vi "ReleaseLock.vi"(7 "Key":T1, 8 "error in (no error)":errorcluster, 11 "Object in":refnum<class "OpenG_Reference_Object.lvclass">) -> (0 "error out":errorcluster, 3 "Object out":refnum<class "OpenG_Reference_Object.lvclass">)   [LabVIEW 2015, in "OpenG_Reference_Object.lvclass"]
doc: "Releases a locked object to allow other parallel threads to access the object. Proper key is required to unlock an object."
uses:
  <userlib>/_OpenG.lib/openg_object/openg_reference_object.llb/OpenG_Reference_Object.lvclass
  <userlib>/_OpenG.lib/openg_object/openg_reference_object.llb/Key.ctl
  <userlib>/_OpenG.lib/openg_object/openg_reference_object.llb/OpenG_Reference_Object.lvclass/OpenG_Reference_Object.ctl
panel:
  # "Please visit http://www.OpenG.org to learn about the\nOpen Source LabVIEW software movement.\n\nNOTICE -- YOU MUST LEAVE THIS NOTICE IN PLACE.  PER THE TERMS OF THE LICENSE BELOW, YOU MAY SUBLICENSE THIS SOFTWARE \nIN ANY WAY THAT DOES NOT CONFLICT WITH THIS LICENSE.\n\n### BSD License (http://www.opensource.org/licenses/bsd-license.php) Begin ###\n\nCopyright (c) 2007, Tomi Maila\nCopyright (c) 2007, Endevo AB\n\n\nAll rights reserved.\n\nRedistribution and use in source and binary forms, with or without modification, are permitted provided that the following conditions are met:\n\n    * Redistributions of source code must retain the above copyright notice, this list of conditions and the following disclaimer.\n    * Redistributions in binary form must reproduce the above copyright notice, this list of conditions and the following disclaimer in the \n       documentation and/or other materials provided with the distribution.\n    * Neither the name of Endevo AB nor the names of the contributors may be used to endorse or promote products derived\n       from this software without specific prior written permission.\n\nTHIS SOFTWARE IS PROVIDED BY THE COPYRIGHT HOLDERS AND CONTRIBUTORS \"AS IS\" AND ANY EXPRESS OR IMPLIED WARRANTIES, \nINCLUDING, BUT NOT LIMITED TO, THE IMPLIED WARRANTIES OF MERCHANTABILITY AND FITNESS FOR A PARTICULAR PURPOSE ARE \nDISCLAIMED. IN NO EVENT SHALL THE COPYRIGHT OWNER OR CONTRIBUTORS BE LIABLE FOR ANY DIRECT, INDIRECT, INCIDENTAL,\n SPECIAL, EXEMPLARY, OR CONSEQUENTIAL DAMAGES (INCLUDING, BUT NOT LIMITED TO, PROCUREMENT OF SUBSTITUTE GOODS OR \nSERVICES; LOSS OF USE, DATA, OR PROFITS; OR BUSINESS INTERRUPTION) HOWEVER CAUSED AND ON ANY THEORY OF LIABILITY, \nWHETHER IN CONTRACT, STRICT LIABILITY, OR TORT (INCLUDING NEGLIGENCE OR OTHERWISE) ARISING IN ANY WAY OUT OF THE USE \nOF THIS SOFTWARE, EVEN IF ADVISED OF THE POSSIBILITY OF SUCH DAMAGE.\n\n### BSD License End ###"
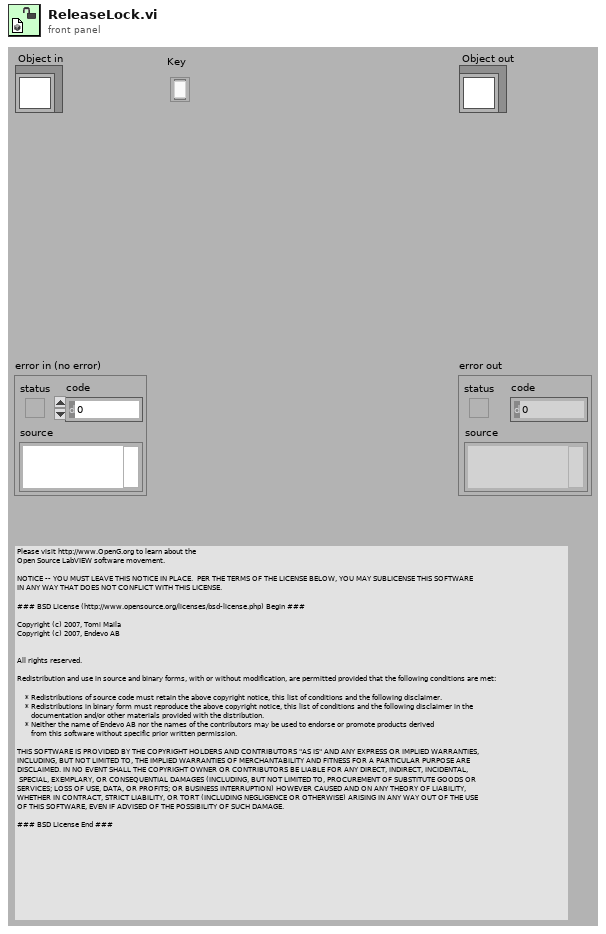
[diagram p1: front panel]
types:
  T1 = typedef "OpenG_Reference_Object.lvclass/Key.ctl" = refnum<k1>
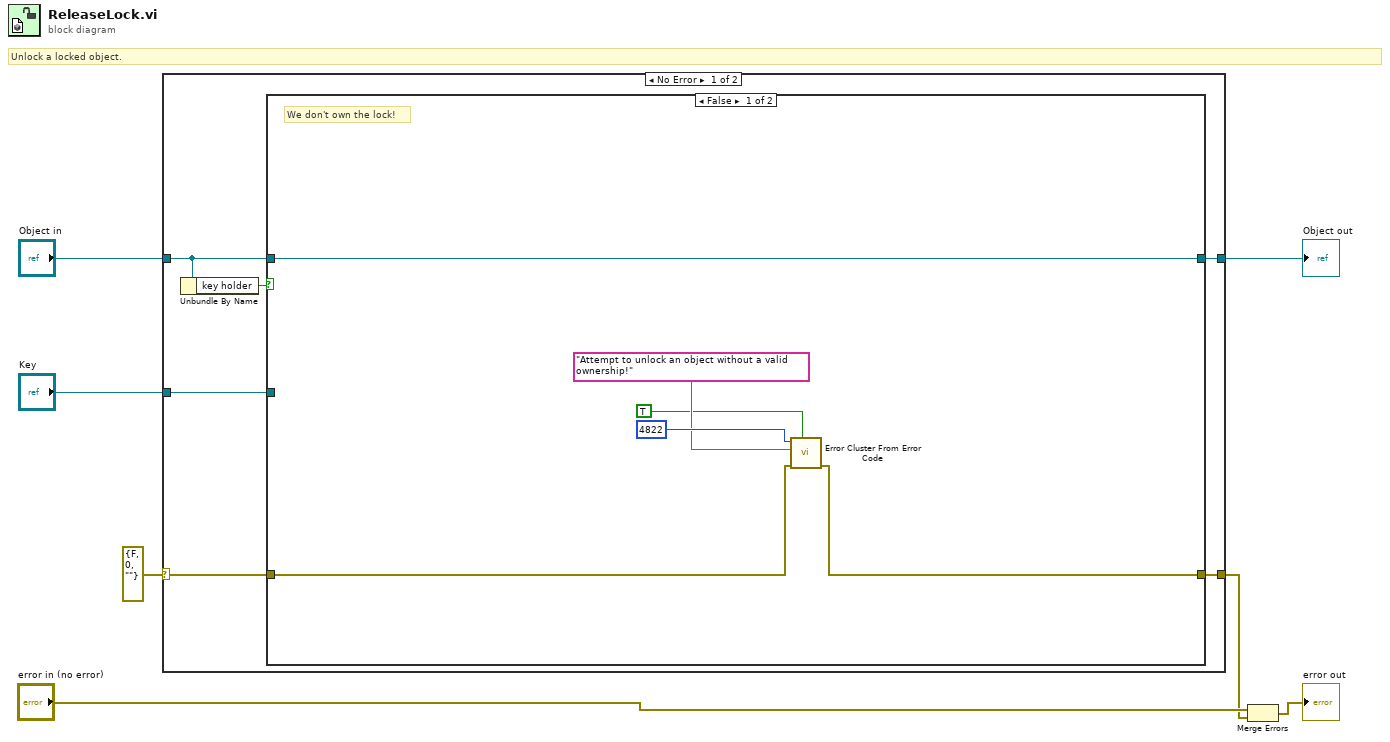
[diagram p0: block diagram]
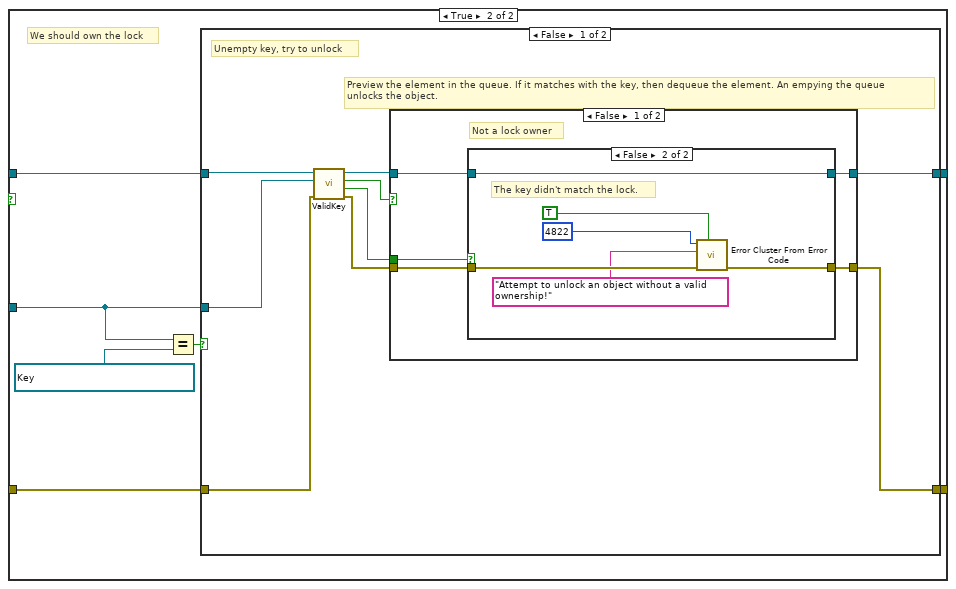
[diagram p2: hidden frame]
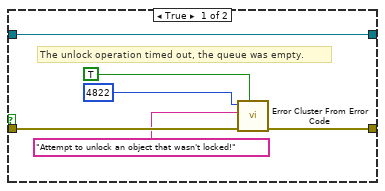
[diagram p3: hidden frame]
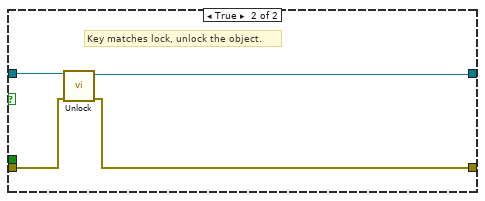
[diagram p4: hidden frame]
diagram:
  # "Unlock a locked object."
  n1 = case shown="No Error" errorcluster {"status"=FALSE, "code"=0, "source"=""} ("error IO") {
    selector: errorcluster {"status"=FALSE, "code"=0, "source"=""} ("error IO") -> [w11 w60]
    tunnel: [w13 w60] -> w2
    tunnel: [w12 w59] -> w6
    tunnel: "Object in" -> [w10 w59]
    tunnel: "Key" -> [w8 _]
    frame No Error {
      n2 = Unbundle By Name(w10) -> ("key holder"=w9:bool)
      n3 = case shown="False" w9 {
        tunnel: [w16 w26] -> w13
        tunnel: [w14 w25] -> w12
        tunnel: w10 -> [w14 w24]
        tunnel: w11 -> [w15 w23]
        tunnel: w8 -> [_ w20]
        frame False {
          # "We don't own the lock!"
          n4 = call <vilib>:"Error Cluster From Error Code.vi"("show call chain? (False)"=TRUE, "error in (no error)"=w15, "error message (\"\")"="Attempt to unlock an object without a valid ownership!" ("source"), "error code (0)"=4822 ("code")) -> ("error out"=w16:errorcluster)  [unwired: 5 in]
        }
        frame True {
          w22 = T1 refnum items=["Open Reference Object Key"] ("Open Reference Object Key")
          # "We should own the lock"
          n5 = Equal?(x=w20, y=w22) -> (x = y?=w21:bool)
          n6 = case shown="False" w21 {
            tunnel: [w35 w57] -> w26
            tunnel: [w34 w58] -> w25
            tunnel: w24 -> [w33 w58]
            tunnel: w23 -> [w30 w57]
            tunnel: w20 -> [w31 _]
            frame False {
              # "Unempty key, try to unlock"
              # "Preview the element in the queue. If it matches with the key, then dequeue the element. An empying the queue\nunlocks the object."
              n7 = call <userlib>:"ValidKey.vi"("error in (no error)"=w30, "Object Key"=w31, "Object in"=w33) -> ("error out"=w29:errorcluster, "timed out?"=w27:bool, "Valid Key?"=w28:bool, "Object out"=w32:refnum<class "OpenG_Reference_Object.lvclass">)  [unwired: 5 in]
              n8 = case shown="False" w28 {
                tunnel: [w37 w53] -> w35
                tunnel: w29 -> [w38 w54]
                tunnel: w32 -> [w40 w56]
                tunnel: [w36 w55] -> w34
                tunnel: w27 -> [w39 _]
                frame False {
                  # "Not a lock owner"
                  n9 = case shown="False" w39 {
                    tunnel: w40 -> [w41 w47]
                    tunnel: w38 -> [w46 w52]
                    tunnel: [w45 w51] -> w37
                    tunnel: [w41 w47] -> w36
                    frame True {
                      # "The unlock operation timed out, the queue was empty."
                      n10 = call <vilib>:"Error Cluster From Error Code.vi"("show call chain? (False)"=TRUE, "error in (no error)"=w46, "error message (\"\")"="Attempt to unlock an object that wasn't locked!" ("source"), "error code (0)"=4822 ("code")) -> ("error out"=w45:errorcluster)  [unwired: 5 in]
                    }
                    frame False {
                      # "The key didn't match the lock."
                      n11 = call <vilib>:"Error Cluster From Error Code.vi"("show call chain? (False)"=TRUE, "error in (no error)"=w52, "error message (\"\")"="Attempt to unlock an object without a valid ownership!" ("source"), "error code (0)"=4822 ("code")) -> ("error out"=w51:errorcluster)  [unwired: 5 in]
                    }
                  }
                }
                frame True {
                  # "Key matches lock, unlock the object."
                  n12 = call <userlib>:"Unlock.vi"("error in (no error)"=w54, "Object in"=w56) -> ("error out"=w53:errorcluster, "Object out"=w55:refnum<class "OpenG_Reference_Object.lvclass">)  [unwired: 8 in]
                }
              }
            }
            frame True {
              # "Empty key, no need to unlock"
            }
          }
        }
      }
    }
    frame Error {
    }
  }
  "Object out" <- w6
  n13 = Merge Errors("error in (no error)", w2) -> (→"error out":errorcluster)
